vi "Calibration_Image_Save.vi"(9 "SN":string, 10 "file":path) -> (1 "error out":errorcluster, 2 "path":path)   [LabVIEW 2017]
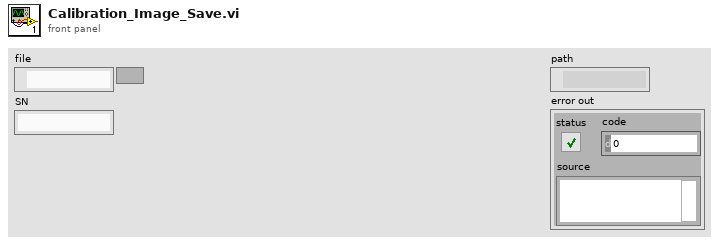
[diagram p1: front panel]
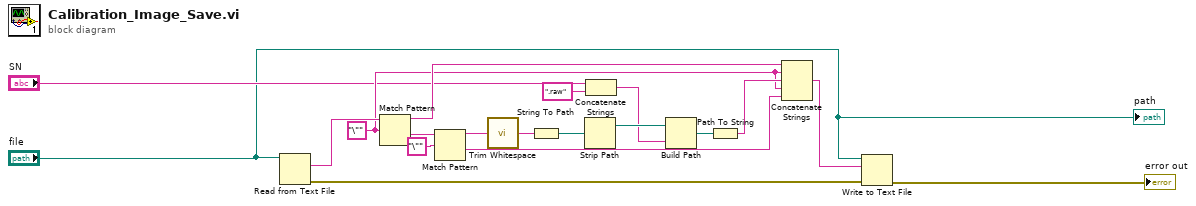
[diagram p0: block diagram]
diagram:
  w6 = "\"" ("regular expression")
  n1 = Read from Text File(file (use dialog)="file") -> (text=w16:string, error out=w19:errorcluster)  [unwired: 3 in, 2 out]
  n2 = Match Pattern(string=w16, regular expression=w6) -> (before substring=w8:string, after substring=w17:string)  [unwired: 1 in, 2 out]
  n3 = Match Pattern(string=w17, regular expression="\"") -> (before substring=w15:string, after substring=w5:string)  [unwired: 1 in, 2 out]
  n4 = call <vilib>:"Trim Whitespace.vi"("string"=w15) -> ("trimmed string"=w14:string)  [unwired: 1 in]
  n5 = String To Path(string=w14) -> (path=w13:path)
  n6 = Strip Path(path=w13) -> (stripped path=w12:path)  [unwired: 1 out]
  n7 = Concatenate Strings("SN", ".raw") -> (w10:string)
  n8 = Build Path(base path=w12, name or relative path=w10) -> (appended path=w9:path)
  n9 = Path To String(path=w9) -> (string=w7:string)
  n10 = Concatenate Strings(w8, w6, w7, w6, w5) -> (w4:string)
  n11 = Write to Text File(file (use dialog)="file", text=w4, error in=w19) -> (error out=→"error out":errorcluster)  [unwired: 1 in, 2 out]
  "path" <- "file"
